vi "miliGAT_subVI.vi"(8 "Error In":errorcluster, 9 "User Input":i32, 10 "?":u16(ring) items=["Dispense, 0.001<n<1E15 uL", "Set Pump Count to Zero", "Print Pump Position Count", "Set Pump Speed (20-160 uL/sec)", "Print Pump Speed", "Stop Pump"], 11 "miliGAT Comm In":refnum<visa-resource-name>="COM6") -> (0 "error out":errorcluster, 2 "Answer":string, 3 "miliGAT Comm Out":refnum<visa-resource-name>)   [LabVIEW 2011]
panel:
  out "bytes read 2":u32
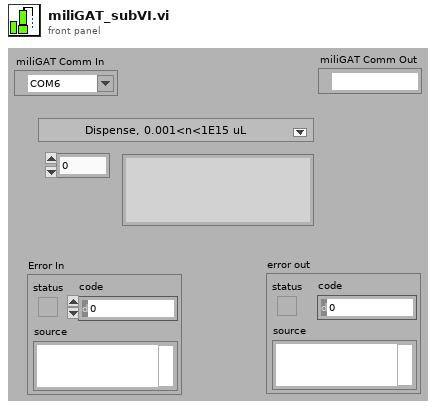
[diagram p1: front panel]
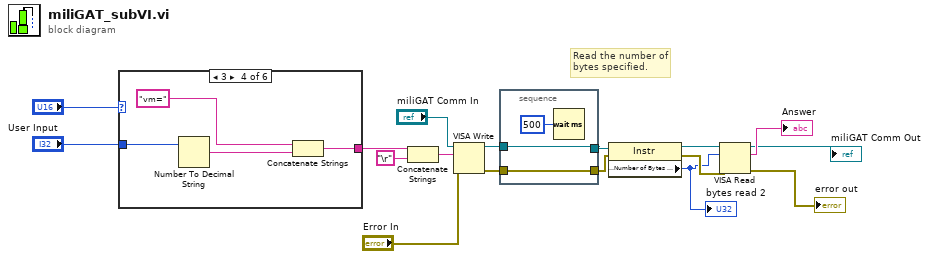
[diagram p0: block diagram]
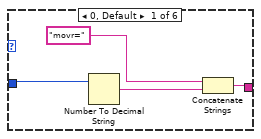
[diagram p2: hidden frame]
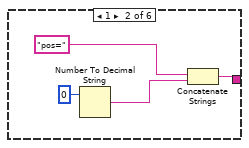
[diagram p3: hidden frame]
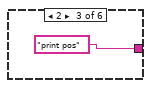
[diagram p4: hidden frame]
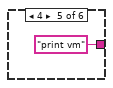
[diagram p5: hidden frame]
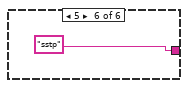
[diagram p6: hidden frame]
diagram:
  # "Read the number of bytes specified."
  n1 = case shown="3" "?" {
    tunnel: [w19 w22 "print pos" w30 "print vm" "sstp"] -> w13
    tunnel: "User Input" -> [w18 _ _ w29 _ _]
    frame 0, Default {
      n2 = Number To Decimal String(number=w18) -> (decimal integer string=w20:string)  [unwired: 1 in]
      n3 = Concatenate Strings("movr=", w20) -> (w19:string)
    }
    frame 1 {
      n4 = Number To Decimal String(number=0) -> (decimal integer string=w25:string)  [unwired: 1 in]
      n5 = Concatenate Strings("pos=", w25) -> (w22:string)
    }
    frame 2 {
    }
    frame 3 {
      n6 = Number To Decimal String(number=w29) -> (decimal integer string=w27:string)  [unwired: 1 in]
      n7 = Concatenate Strings("vm=", w27) -> (w30:string)
    }
    frame 4 {
    }
    frame 5 {
    }
  }
  n8 = Concatenate Strings(w13, "\r") -> (w6:string)
  n9 = VISA Write(VISA resource name="miliGAT Comm In", write buffer=w6, error in (no error)="Error In") -> (VISA resource name out=w12:refnum<visa-resource-name>, error out=w11:errorcluster)  [unwired: 1 out]
  n10 = stacked-sequence {
    tunnel: w12 -> [w35]
    tunnel: w11 -> [w34]
    tunnel: [w35] -> w8
    tunnel: [w34] -> w7
    frame #0 {
      n11 = Wait (ms)(milliseconds to wait=u32 500) -> ()  [unwired: 1 out]
    }
  }
  n12 = property class="Instr"(reference=w8, error in=w7) -> (reference out=w10:refnum<visa-resource-name>, error out=w9:errorcluster, "Serial Settings:Number of Bytes at Serial Port"=w4:u32)
  "bytes read 2" <- w4
  n13 = VISA Read(VISA resource name=w10, byte count=w4, error in (no error)=w9) -> (VISA resource name out=→"miliGAT Comm Out":refnum<visa-resource-name>, read buffer=→"Answer":string, error out=→"error out":errorcluster)  [unwired: 1 out]
